vi "string2hexcmd.vi"(0 "String comand":string) -> (1 "hex comand":string, 2 "byte count":u32)   [LabVIEW 2010]
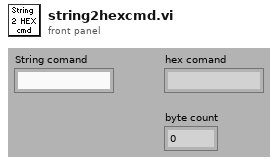
[diagram p1: front panel]
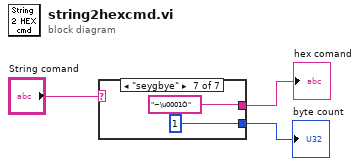
[diagram p0: block diagram]
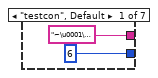
[diagram p2: hidden frame]
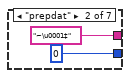
[diagram p3: hidden frame]
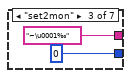
[diagram p4: hidden frame]
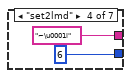
[diagram p5: hidden frame]
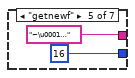
[diagram p6: hidden frame]
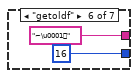
[diagram p7: hidden frame]
diagram:
  n1 = case shown="\"seygbye\"" "String comand" {
    tunnel: [6 0 0 6 16 16 1] -> w3
    tunnel: ["~\u0001\u0000" "~\u0001‡" "~\u0001‰" "~\u0001i" "~\u0001…" "~\u0001" "~\u0001Ò"] -> w2
    frame "testcon", Default {
    }
    frame "prepdat" {
    }
    frame "set2mon" {
    }
    frame "set2lmd" {
    }
    frame "getnewf" {
    }
    frame "getoldf" {
    }
    frame "seygbye" {
    }
  }
  "byte count" <- w3
  "hex comand" <- w2
